vi "GetCommands.vi"(8 "error in (no error)":errorcluster, 11 "reference in":refnum<class "RemoteControl.lvclass">) -> (0 "error out":errorcluster, 1 "OfCommands":refnum<class "Command.lvclass">[](array[class]), 2 "OnCommands":refnum<class "Command.lvclass">[](array[class]), 3 "reference out":refnum<class "RemoteControl.lvclass">)   [LabVIEW 2012, in "RemoteControl.lvclass"]
uses:
  RemoteControl.lvclass
  Command_class/Command.lvclass
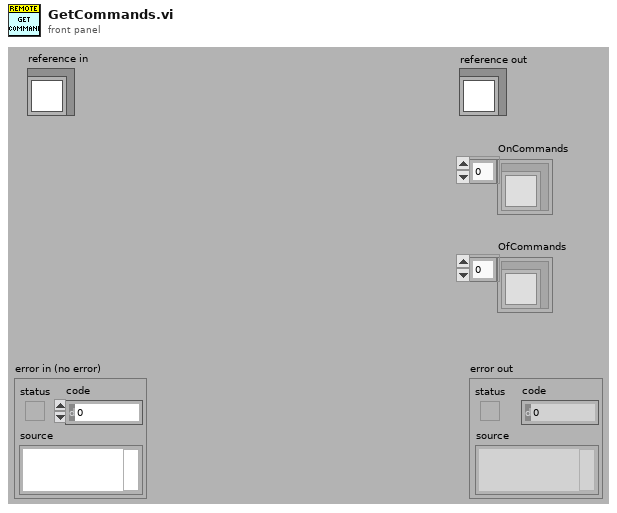
[diagram p1: front panel]
types:
  T1 = typedef "RemoteControl.lvclass/ObjectAttributes.ctl" = cluster{"OnCommands":refnum<class "Command.lvclass">[], "OffCommands":refnum<class "Command.lvclass">[], "UndoCommand":refnum<class "Command.lvclass">}
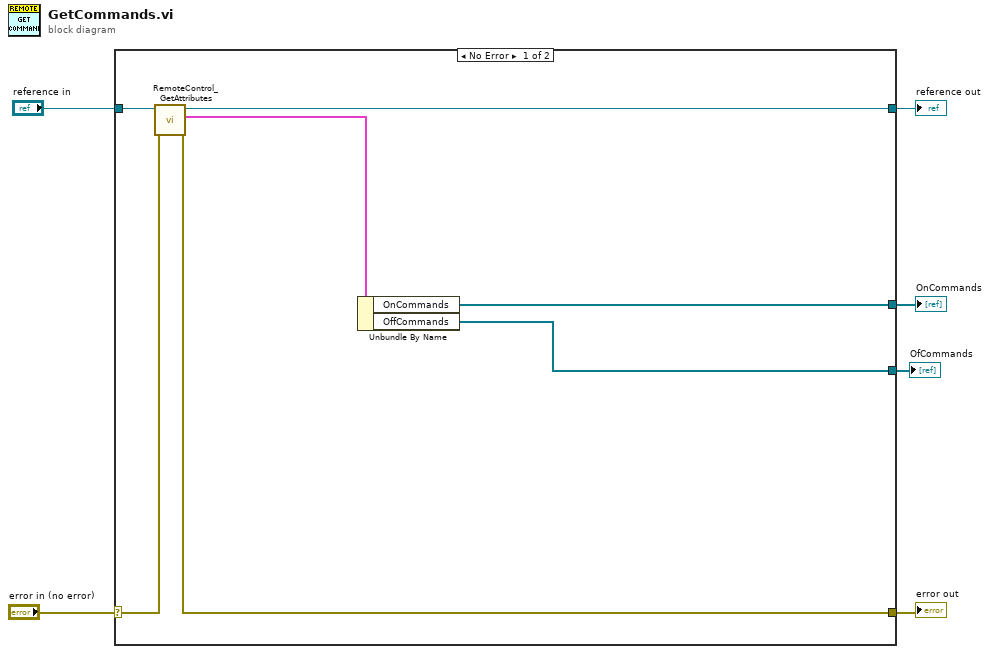
[diagram p0: block diagram]
diagram:
  n1 = case shown="No Error" "error in (no error)" {
    selector: "error in (no error)" -> [w13 w15]
    tunnel: [w11 w15] -> w5
    tunnel: [w9 w14] -> w3
    tunnel: "reference in" -> [w10 w14]
    tunnel: [w8 _] -> w2
    tunnel: [w7 _] -> w1
    frame No Error {
      n2 = call "RemoteControl_GetAttributes.vi"("error in (no error)"=w13, "reference in"=w10) -> ("error out"=w11:errorcluster, "Data"=w12:T1, "reference out"=w9:refnum<class "RemoteControl.lvclass">)  [unwired: 6 in, 1 out]
      n3 = Unbundle By Name(w12) -> ("OnCommands"=w8:refnum<class "Command.lvclass">[], "OffCommands"=w7:refnum<class "Command.lvclass">[])
    }
    frame Error {
    }
  }
  "error out" <- w5
  "reference out" <- w3
  "OnCommands" <- w2
  "OfCommands" <- w1
